vi "ReadAll.vi"(0 "object in":refnum<class "CoriFlowBFS1Plus.lvclass">, 2 "Buffer Values?":bool=TRUE, 5 "error in (no error)":errorcluster) -> (14 "object out":refnum<class "CoriFlowBFS1Plus.lvclass">, 16 "Coriolis Data":T1, 19 "error out":errorcluster)   [LabVIEW 2021, in "CoriFlowBFS1Plus.lvclass"]
uses:
  CoriFlowBFS1Plus.lvclass
  CoriFlowBFS1Plus.lvclass/CoriFlowBFS1Plus.ctl
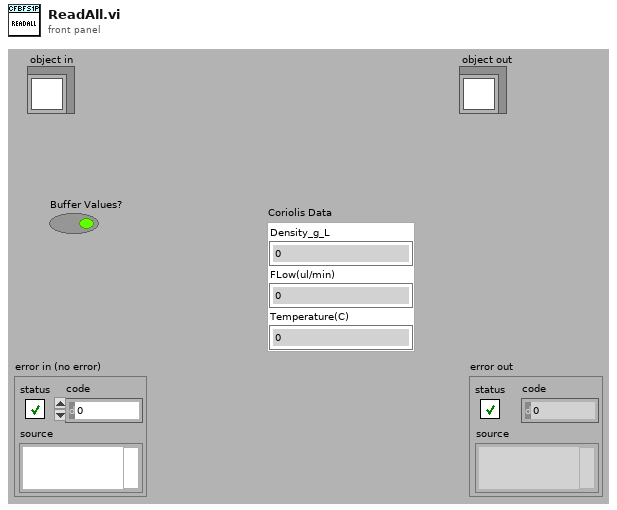
[diagram p1: front panel]
types:
  T1 = cluster{"Density_g_L":sgl, "FLow(ul/min)":sgl, "Temperature(C)":sgl}
  T2 = cluster{"Cluster":cluster{"Density_g_L":sgl, "FLow(ul/min)":sgl, "Temperature(C)":sgl}, "current time":timestamp}
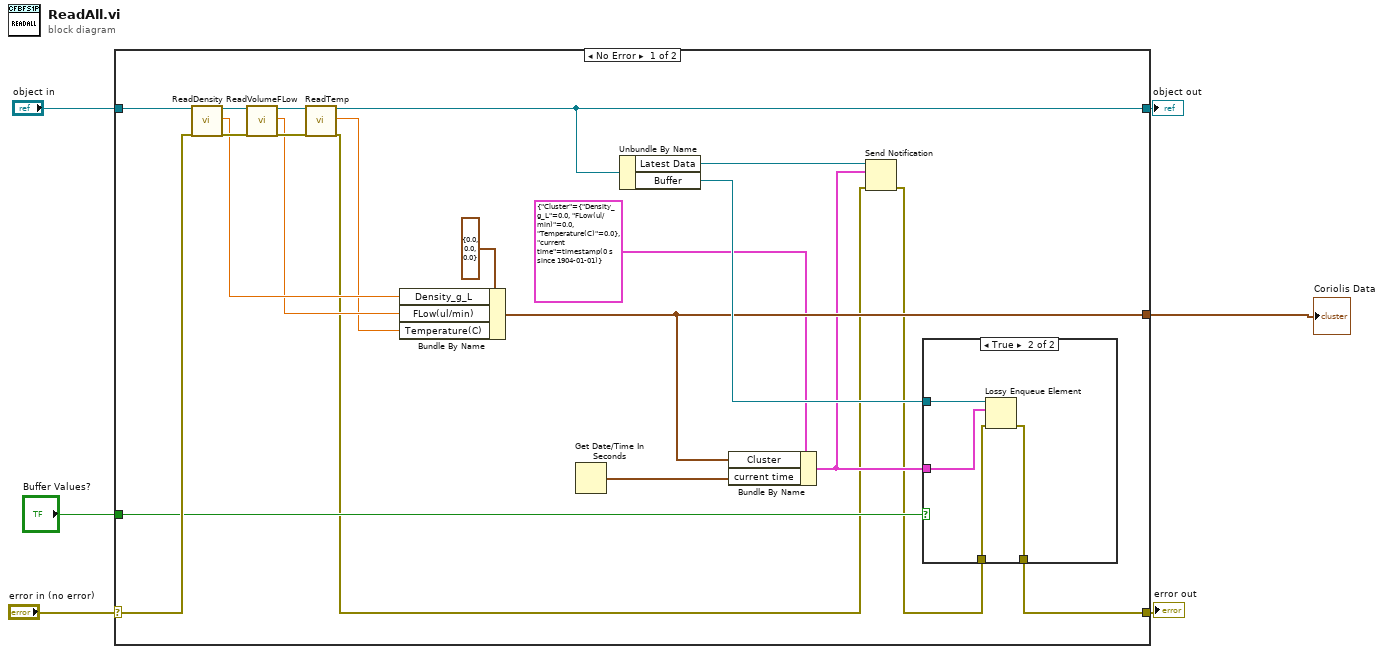
[diagram p0: block diagram]
diagram:
  n1 = case shown="No Error" "error in (no error)" {
    selector: "error in (no error)" -> [w22 w34]
    tunnel: [w15 w34] -> w5
    tunnel: [w17 w33] -> w3
    tunnel: "object in" -> [w25 w33]
    tunnel: [w13 _] -> w2
    tunnel: "Buffer Values?" -> [w10 _]
    frame No Error {
      n2 = call-dynamic "ReadDensity.vi"("object in"=w25, "error in (no error)"=w22) -> ("object out"=w27:refnum<class "CoriFlowBFS1Plus.lvclass">, "Density_g_L"=w20:sgl, "error out"=w24:errorcluster)  [unwired: 15 in]
      n3 = call-dynamic "ReadVolumeFLow.vi"("object in"=w27, "error in (no error)"=w24) -> ("object out"=w26:refnum<class "CoriFlowBFS1Plus.lvclass">, "FLow(ul/min)"=w19:sgl, "error out"=w23:errorcluster)  [unwired: 15 in]
      n4 = call-dynamic "ReadTemp.vi"("object in"=w26, "error in (no error)"=w23) -> ("object out"=w17:refnum<class "CoriFlowBFS1Plus.lvclass">, "Temperature(C)"=w18:sgl, "error out"=w8:errorcluster)  [unwired: 15 in]
      n5 = Bundle By Name(cluster=T1 {"Density_g_L"=0.0, "FLow(ul/min)"=0.0, "Temperature(C)"=0.0} ("Cluster"), "Density_g_L"=w20, "FLow(ul/min)"=w19, "Temperature(C)"=w18) -> (w13:T1)
      n6 = Get Date/Time In Seconds() -> (seconds since 1Jan1904=w11:timestamp)
      n7 = Unbundle By Name(w17) -> ("Latest Data"=w14:refnum<notifier>, "Buffer"=w16:refnum<queue>)
      n8 = Bundle By Name(cluster=T2 {"Cluster"={"Density_g_L"=0.0, "FLow(ul/min)"=0.0, "Temperature(C)"=0.0}, "current time"=timestamp(0 s since 1904-01-01)} ("element"), "Cluster"=w13, "current time"=w11) -> (w9:T2)
      n9 = Send Notification(notification=w9, notifier=w14, error in (no error)=w8) -> (error out=w7:errorcluster)  [unwired: 1 out]
      n10 = case shown="True" w10 {
        tunnel: w16 -> [_ w32]
        tunnel: w7 -> [w28 w31]
        tunnel: [w28 w30] -> w15
        tunnel: w9 -> [_ w29]
        frame False {
        }
        frame True {
          n11 = Lossy Enqueue Element(queue=w32, element=w29, error in (no error)=w31) -> (error out=w30:errorcluster)  [unwired: 3 out]
        }
      }
    }
    frame Error {
    }
  }
  "error out" <- w5
  "object out" <- w3
  "Coriolis Data" <- w2
